vi "Initialize Resources.vi"(7 "CD Name":string, 8 "error in":errorcluster, 10 "CDAPI in":refnum<class "CustomDeviceAPI.lvclass">, 11 "Template in":refnum<class "Template.lvclass">) -> (0 "error out":errorcluster, 3 "Template out":refnum<class "Template.lvclass">)   [LabVIEW 2026, in "Template Plugin.lvlib" / "Template.lvclass"]
uses:
  Template.lvclass
  Template.lvclass/Template.ctl
  <userlib>/CustomDeviceInterfaces_v1.lvlibp/custom-device-express-framework/Source/Custom Device Interfaces/CustomDeviceAPI/CustomDeviceAPI.lvclass
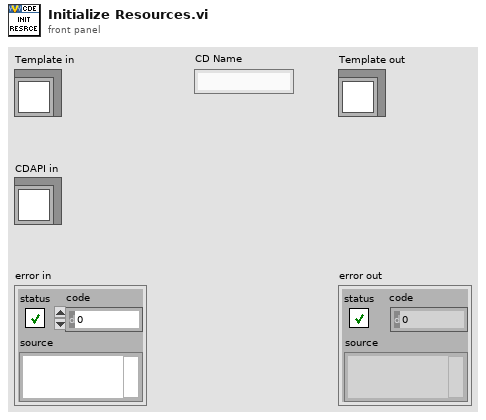
[diagram p1: front panel]
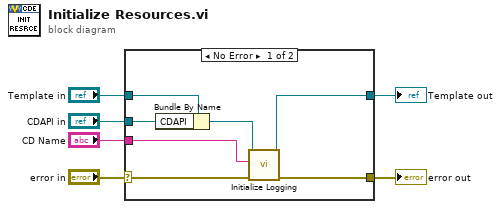
[diagram p0: block diagram]
diagram:
  n1 = case shown="No Error" "error in" {
    selector: "error in" -> [w13 w15]
    tunnel: [w12 w15] -> w5
    tunnel: [w11 w14] -> w3
    tunnel: "Template in" -> [w9 w14]
    tunnel: "CD Name" -> [w10 _]
    tunnel: "CDAPI in" -> [w8 _]
    frame No Error {
      n2 = Bundle By Name(cluster=w9, "CDAPI"=w8) -> (w7:refnum<class "Template.lvclass">)
      n3 = call "Initialize Logging.vi"("error in"=w13, "Plugin Name"=w10, "Template in"=w7) -> ("error out"=w12:errorcluster, "Template out"=w11:refnum<class "Template.lvclass">)  [unwired: 7 in]
    }
    frame Error {
    }
  }
  "error out" <- w5
  "Template out" <- w3
